vi "Big_LED_control.vi"() -> ()   [LabVIEW 2018]
uses:
  <instrlib>/niDCPower/nidcpower.llb/niDCPower Source Mode.ctl
  <instrlib>/niDCPower/nidcpower.llb/niDCPower Output Function.ctl
  AT lib/AmateurStepperMotor.dll
  <instrlib>/niDMM/nidmm.llb/niDMM Function.ctl
  <instrlib>/niDMM/nidmm.llb/niDMM Resolution in Digits.ctl
  <vilib>/Instr/_visa.llb/VISA Configure Serial Port (Instr).vi
  <instrlib>/niDMM/nidmm.llb/niDMM Configure Measurement Digits.vi
panel:
  in  "Tab Control 2":enum32{"Шаговик и офир", "Служебная область"}(tab)
  in  "milliseconds to wait":u32=1000
  in  "Go To":dbl
  out "Ophir 1 Char":dbl(graph)=0.02
  in  "DecelerationTime, s":dbl=0.3
  in  "AccelerationTime, s":dbl=0.3
  in  "HoldOn":bool
  in  "Ophir 1 units":string(combo)="1000" caption="Units"
  out "Ophir 1 Over Range":bool caption="Over Range"
  out "Ophir 1 Optical Power":dbl=0.02 caption="Power" format="%#_4g"
  out "Ophir 1 MAX":dbl=0.030000000000000002 caption="MAX" format="%#_5g"
  in  "Ophir 1 Clear":bool caption="Clear"
  in  "StepMultiplicationFactor":dbl=50.0
  in  "StepDivisor":i32(ring)=8 items=["D1"=1, "D2"=2, "D4"=4, "D8"=8, "D16"=16, "D32"=32]
  in  "Speed":dbl=250.0
  in  "Погнали!":bool
  in  "Стоп GoTo":bool
  out "Готово":bool
  out "Position":dbl
  in  "Ophir 1 Info":u16(ring)=1 caption="Info" items=["Device : JUNO; s/n:903793", "Head : PD300R-3W   ; s/n:779628"]
  in  "new pos":dbl
  in  "set pos":bool
  out "Device Response":string="*\n"
  in  "Ophir 1 usb channel":i16 caption="usb channel"
  out "Ophir 1 dup Visa Session":refnum<visa-resource-name>="USB0::0x0BD3::0x0777::NI-VISA-60004::RAW" caption="dup Visa Session"
  in  "Ophir 1 Baud Rate (3:9600)":i16(ring)=3 caption="Baud Rate (3:9600)" items=["300", "1200", "4800", "9600", "19200", "38400"]
  out "Ophir 1 Real Optical Power":dbl=2e-05 format="%.6e"
  in  "Ophir 1 GPIB Address (10)":string="10" caption="GPIB Address (10)"
  in  "Ophir 1 Port Number (default 2)":i16=1 caption="Port Number (default 2)" min=0 max=20
  in  "Ophir 1 Select Communication Protocol":u16(ring) caption="Select Communication Protocol" items=["USB", "RS232", "GPIB"]
  out "Ophir 1 error out":errorcluster caption="error out"
  in  "Ophir 1 error in (no error)":errorcluster caption="error in (no error)"
  in  "Ophir 1 Wait":u32=100 caption="Wait"
  out "IsOpen":bool=TRUE
  out "Ophir 1 Initialization":bool=TRUE caption="Initialization"
  in  "Tab Control":T1(tab)
  in  "POWER":bool
  in  "Стоп":bool=TRUE
  in  "Resource Name":refnum<k15>="PXI1Slot2" caption="Источник питания"
  in  "Амперметр":refnum<k15>="PXI1Slot4" caption="NI DMM 1"
  in  "V_MB, V":dbl=6.0 caption="voltage level" min=0.0 max=6.0 format="%_6p"
  in  "curlim_V_MB, A":dbl=0.3 caption="current limit" format="%_6p"
  out "chart_0":dbl(graph)=-0.00019003121552656476 caption="Waveform Chart 5"
  in  "voltlim_I_LED, V":dbl=2.1 caption="current limit" min=0.01 format="%_6p"
  in  "I_LED, A":dbl=0.010000000000000002 caption="voltage level" format="%_6p"
  out "chart_1":dbl(graph)=-0.00011794146773492402 caption="Waveform Chart 5"
  out "Current Char":dbl(graph)=0.004513189196586609
  in  "Arduino":refnum<visa-resource-name>="COM14"
  in  "Сегменты":bool[](array[boolean])=[FALSE, FALSE, FALSE, FALSE, FALSE, FALSE, FALSE, FALSE, FALSE, FALSE, FALSE, FALSE, FALSE, FALSE, FALSE, FALSE, FALSE, FALSE]
  in  "Вольтметр":refnum<k15>="PXI1Slot5" caption="NI DMM 1"
  out "Voltage Char":dbl(graph)=0.015767553821206093
  in  "Port Name":string="COM8" caption="Порт шаговика"
  in  "wave_lenght":string="600"
  in  "Промер":bool caption="Промер сегмента"
  in  "NI DMM 1 Voltage Range 4":string(combo)="-1" caption="Range"
  in  "NI DMM 1 units 4":string(combo)="1" caption="Units"
  out "Voltage":dbl=0.015767553821206093 format="%_6g"
  in  "NI DMM 1 Current Range 3":string(combo)="1" caption="Range"
  in  "NI DMM 1 units 3":string(combo)="1000" caption="Units"
  out "Current":dbl=0.004513189196586609 format="%_6g"
  out "voltmes_V_MB, V":dbl=-0.00019003121552656476 caption="measurement" format="%_6g"
  out "curmes_V_MB, A":dbl=4.978853713564661e-05 caption="measurement" format="%_6g"
  out "curmes_I_LED, A":dbl=4.978853713564661e-05 caption="measurement" format="%_6g"
  out "voltmes_I_LED, V":dbl=-0.00011794146773492402 caption="measurement" format="%_6g"
  out "Разряд":dbl
  out "+/-":bool
  out "Power off":bool=TRUE
  in  "Command":string="Cathode"
  in  "Записать":bool
  out "measure output \nfile refnum":refnum<file>
  out "Voltage, V":dbl=0.015767553821206093 caption="Measurement" format="%.5f"
  out "Current, A":dbl=4.513189196586609e-06 caption="Measurement" format="%.5f"
  out "Тип индикатора":string="Cathode"
  out "chart_2":dbl(graph)=-0.000179732680132088
  in  "V_RES, V":dbl caption="voltage level" format="%_6p"
  out "curmes_V_RES, A":dbl=5.996099535583298e-05 caption="measurement" format="%_6g"
  in  "curlim_V_RES, A":dbl=0.1 caption="current limit" min=0.01 format="%_6p"
  in  "measure path":path=path "C:/Users/user/Desktop/МСП/LabVIEW/LED_CONTROL_big_LED_ophir_24.12.24_1/Logs"
  out "Enum":enum16{"Exit", "4", "Промер", "2", "1"}(ring)
  out "№ об-ца":dbl=1.0
  out "Темп-ра":dbl=1.0
  out "Сегмент":string
  out "voltmes_V_RES, V":dbl=-0.000179732680132088 caption="measurement" format="%_6g"
  in  "current level range":dbl=0.001 format="%#.6p"
  # "При первом запуске  есть ошика при инициализации шаговика.\nПри втором запуске обишки нет, делать ничего не нужно.\n\nПоговорить с Артемом"
  # "Шаговик"
  # "Офир"
  # "Шаговик"
  # "Офир"
  # "position - это значение абсолютное"
  # "j"
  # "c"
  # "d"
  # "e"
  # "g"
  # "h"
  # "a"
  # "b"
  # "f"
  # "k"
  # "L"
  # "m"
  # "n"
  # "p"
  # "dp"
  # "all"
  # "V_MB 5 В\nогрничение 300 м\n\nV_LED 2,1 В\nограничение 200 м"
  # "единицы мА\nrange 1 А"
  # "1. каждый сегмент включаем по отдельности, резистором постраиваем ток до 10 мА\n2. напряжение V_LED при этом не меняется\n3. в такоом положении промеряем сегменты по отдельности\n4. для промера всего индикатора сразу подстраиваем напряжение при неизменном положении резисторов\n5. ток всех индикаторов = ток одного сегмента (10 мА) * число сегментов (15)\n6. добиваемся этого увеличением V_LED"
  # "единицы В\nrange AUTO"
  # "регклировка суммарного тока через индикатор"
  # "24.063\n\n     I          U\n20 мА  1.3 В\n20 мА  1.4 В\n 7 мА   1.15 В"
  # "24.064\n\n     I          U\n10 мА  2 В\n10 мА  2.15 В\n 7 мА   1.9 В"
  # "автоматизировать подбор напряжения по известному максимальному напряжению и току. ОС по току сегмента"
  # "Р1:  +25°C\nР2:  - 60°C\nР3:  +85°C"
  # "регулировать ток в зависимости от температуры.\nс ростом температуры растет ток.\nпид-регулятор??"
  # "0. ввести номер образца\n1. включить нужный сегмент\n2. ввести его в поле справа\n3. вести температуру в поле слева\n4. нажать кнопку \"промер сегмента\""
  # "\"опрашивать кнопки не чаще, чем раз в секунду. сейчас кликать можно чаще, они загорятся, но ничего не произойдет\""
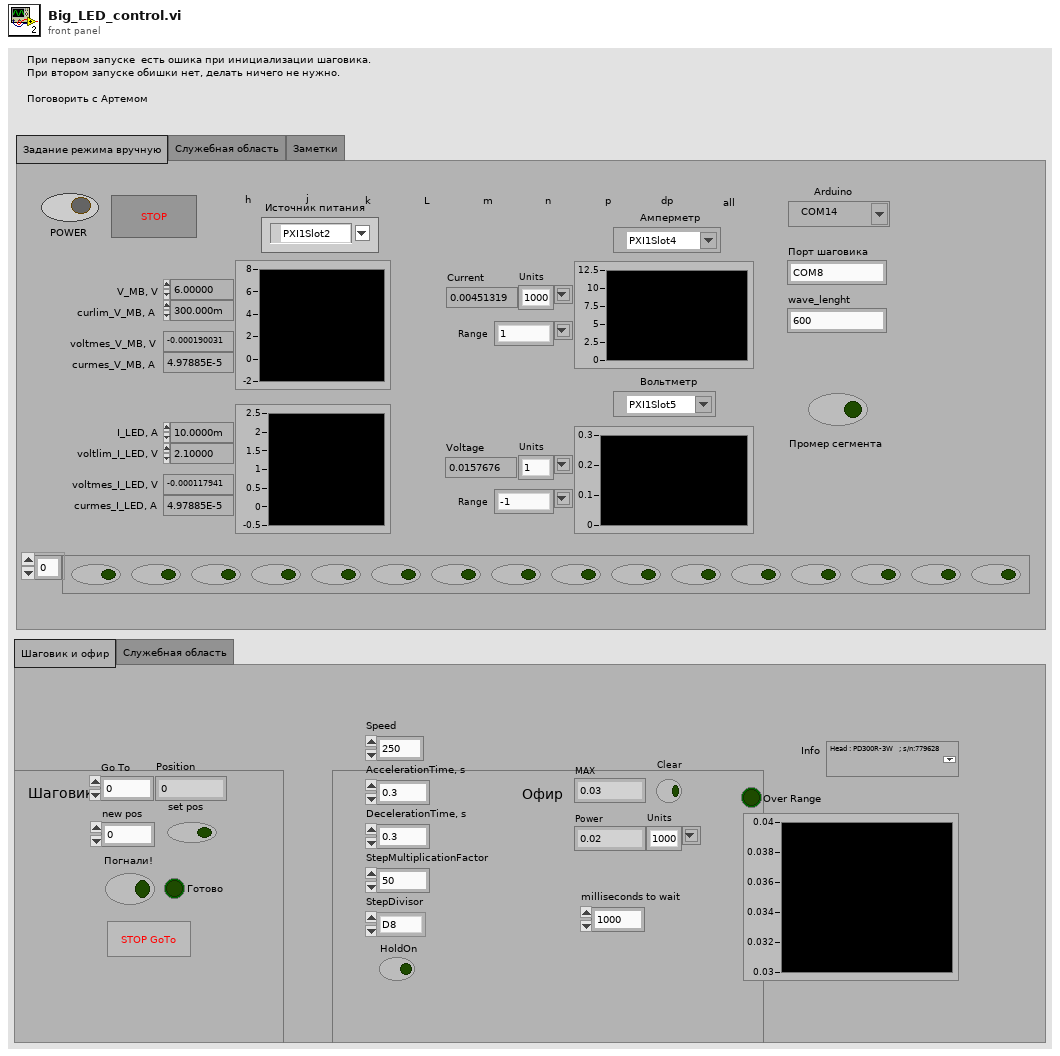
[diagram p1: front panel]
types:
  T1 = enum32{"Задание режима вручную", "Служебная область", "Заметки"}
  T2 = enum16{"open", "replace", "create", "open or create", "replace or create", "replace or create with confirmation"}
  T3 = typedef "niDCPower Output Function.ctl" = i32
  T4 = typedef "niDCPower Source Mode.ctl" = i32
  T5 = typedef "niDMM Function.ctl" = enum16{"DC Volts", "AC Volts", "DC Current", "AC Current", "2-wire Resistance", "4-wire Resistance", "Diode", "Frequency", "Period", "AC Volts DC Coupled", "Capacitance", "Inductance", "Temperature"}
  T6 = typedef "niDMM Resolution in Digits.ctl" = dbl
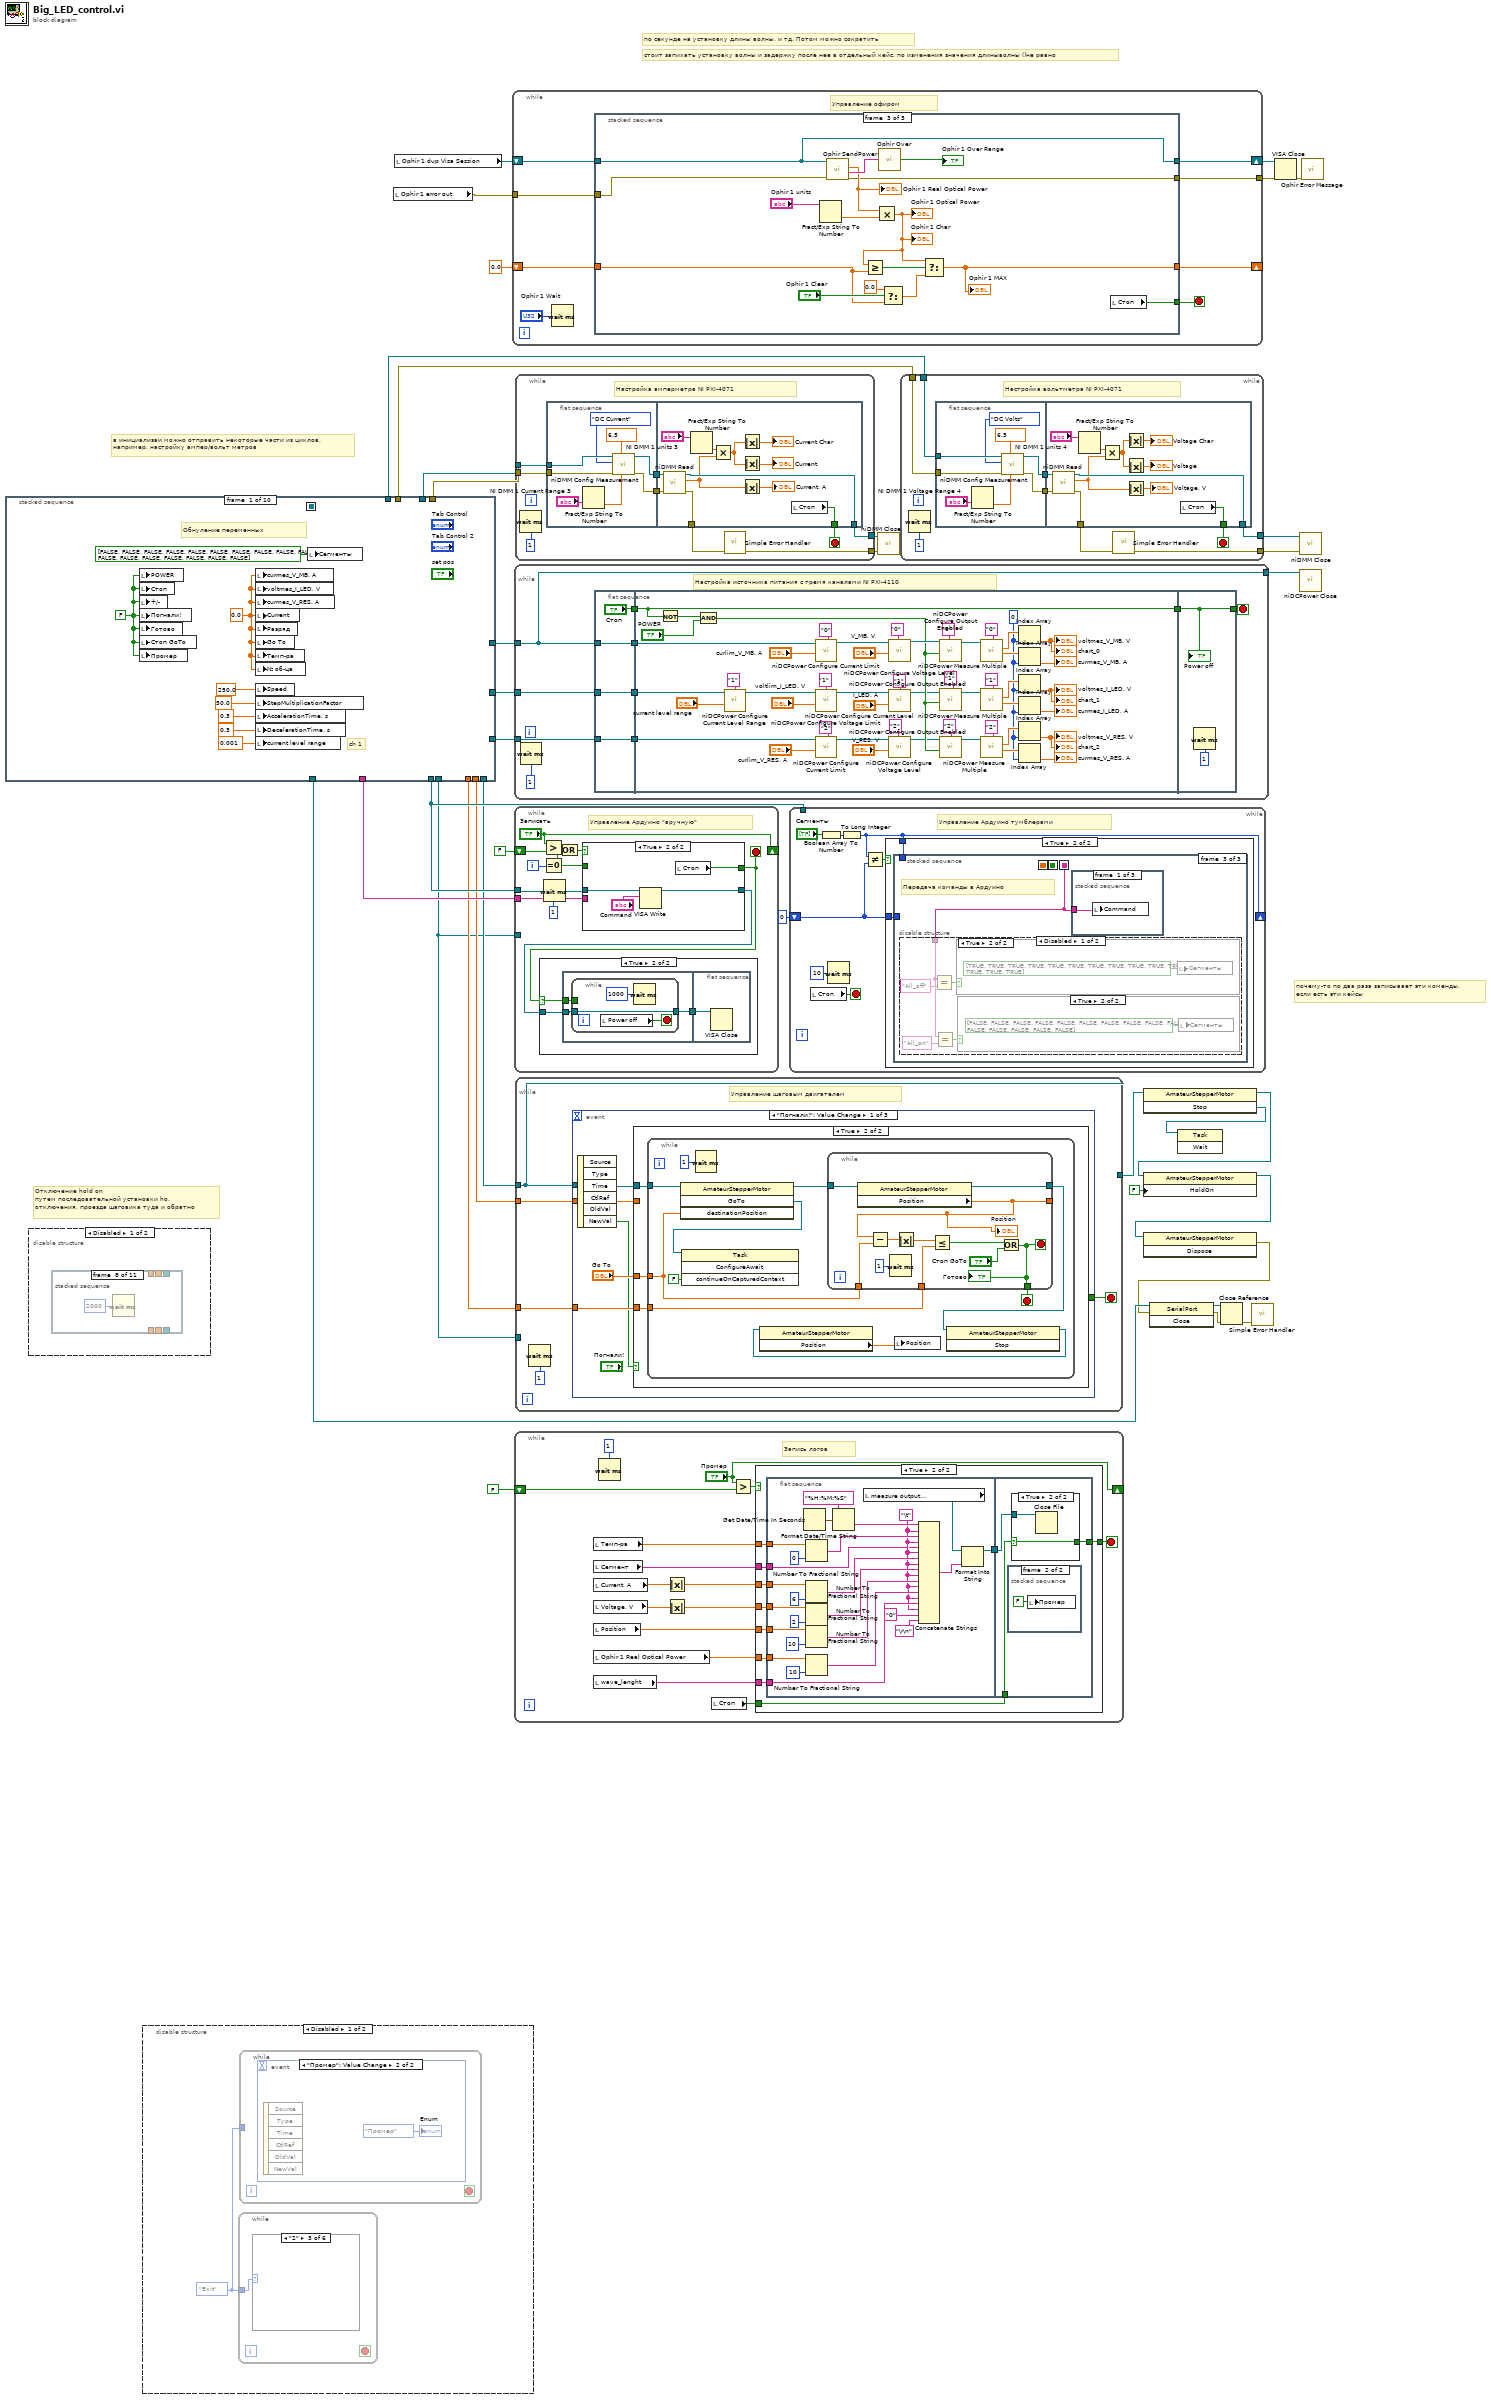
[diagram p0: block diagram]
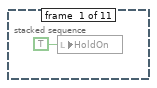
[diagram p2: hidden frame]
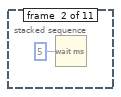
[diagram p3: hidden frame]
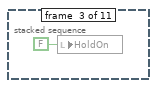
[diagram p4: hidden frame]
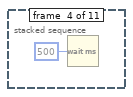
[diagram p5: hidden frame]
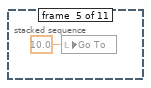
[diagram p6: hidden frame]
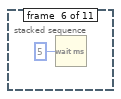
[diagram p7: hidden frame]
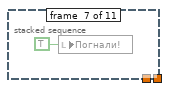
[diagram p8: hidden frame]
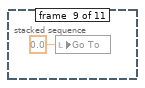
[diagram p9: hidden frame]
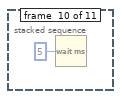
[diagram p10: hidden frame]
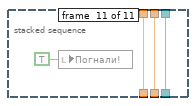
[diagram p11: hidden frame]
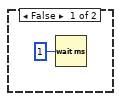
[diagram p13: hidden frame]
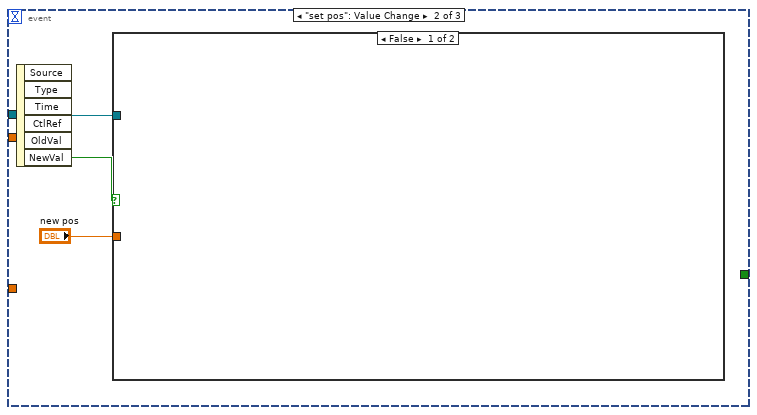
[diagram p14: hidden frame]
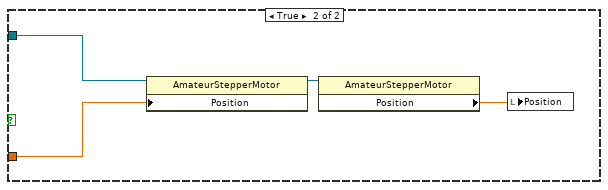
[diagram p15: hidden frame]
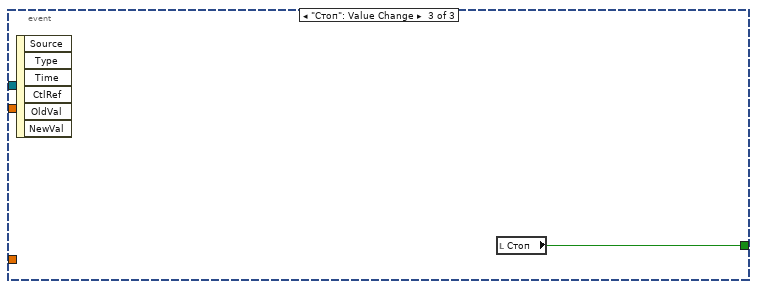
[diagram p16: hidden frame]
diagram:
  # "почему-то по два раза записывает эти коменды,\nесли есть эти кейсы"
  # "Отключение hold on\nпутем последовательной установки ho, \nотключения, проезда шаговика туда и обратно"
  # "в инициализаи можно отправить некоторые части из циклов.\nнапример, настройку ампер/вольт метров"
  # "стоит запихать установку волны и задержку после нее в отдельный кейс, по изменения значения длиныволны ()не равно"
  # "по секунде на установку длины волны, и тд. Потом можно сократить"
  n1 = stacked-sequence {
    seq-local: [_ _ _ _ _ _ w107 _ _ _] -> [_ _ _ _ _ _ _ w116 _ _]
    tunnel: [_ _ _ w54 _ _ _ _ _ _] -> w25
    tunnel: [_ w48 _ _ _ _ _ _ _ _] -> w37
    tunnel: [_ w47 _ _ _ _ _ _ _ _] -> w36
    tunnel: [_ _ _ _ w74 _ _ _ _ _] -> w33
    tunnel: [_ _ _ _ _ _ _ _ w122 _] -> w32
    tunnel: [_ _ w51 _ _ _ _ _ _ _] -> w31
    tunnel: [_ _ w50 _ _ _ _ _ _ _] -> w30
    tunnel: [_ _ _ _ _ _ _ w119 _ _] -> w2
    tunnel: [_ _ _ _ _ _ _ w117 _ _] -> w3
    tunnel: [_ _ _ _ _ _ _ w118 _ _] -> w4
    tunnel: [_ _ _ _ _ _ w97 _ _ _] -> w19
    tunnel: [_ _ _ w53 _ _ _ _ _ _] -> w7
    tunnel: [_ _ _ w52 _ _ _ _ _ _] -> w5
    tunnel: [_ _ _ _ _ _ _ _ _ w123] -> w1
    frame #0 {
      w38 = 0.0 ("currentmes_2")
      w39 = FALSE ("Стоп")
      # "ch 1"
      # "Обнуление переменных"
      n2 = local write "POWER"(w39) -> ()
      n3 = local write "Стоп"(w39) -> ()
      n4 = local write "+/-"(w39) -> ()
      n5 = local write "Погнали!"(w39) -> ()
      n6 = local write "Готово"(w39) -> ()
      n7 = local write "Стоп GoTo"(w39) -> ()
      n8 = local write "Промер"(w39) -> ()
      n9 = local write "curmes_V_MB, A"(w38) -> ()
      n10 = local write "voltmes_I_LED, V"(w38) -> ()
      n11 = local write "curmes_V_RES, A"(w38) -> ()
      n12 = local write "Current"(w38) -> ()
      n13 = local write "Разряд"(w38) -> ()
      n14 = local write "Go To"(w38) -> ()
      n15 = local write "Темп-ра"(w38) -> ()
      n16 = local write "№ об-ца"(w38) -> ()
      n17 = local write "Speed"(250.0 ("Speed")) -> ()
      n18 = local write "StepMultiplicationFactor"(50.0 ("StepMultiplicationFactor")) -> ()
      n19 = local write "AccelerationTime, s"(0.3 ("AccelerationTime, s")) -> ()
      n20 = local write "DecelerationTime, s"(0.3 ("DecelerationTime, s")) -> ()
      n21 = local write "current level range"(0.001 ("current level range")) -> ()
      n22 = local write "Сегменты"(bool[] [FALSE, FALSE, FALSE, FALSE, FALSE, FALSE, FALSE, FALSE, FALSE, FALSE, FALSE, FALSE, FALSE, FALSE, FALSE, FALSE, FALSE, FALSE] ("Сегменты")) -> ()
    }
    frame #1 {
      # "Инициализация амперметра"
      n23 = call <instrlib>:"niDMM Initialize.vi"("Instrument Descriptor"="Амперметр") -> ("error out"=w48:errorcluster, "instrument handle out"=w47:refnum<k15>)  [unwired: 9 in]
    }
    frame #2 {
      # "Инициализация вольтметра"
      n24 = call <instrlib>:"niDMM Initialize.vi"("Instrument Descriptor"="Вольтметр") -> ("error out"=w50:errorcluster, "instrument handle out"=w51:refnum<k15>)  [unwired: 9 in]
    }
    frame #3 {
      w59 = T3 1006 items=["DC Voltage"=1006, "DC Current"=1007, "Pulse Voltage"=1049, "Pulse Current"=1050] ("output function")
      w63 = T3 1007 items=["DC Voltage"=1006, "DC Current"=1007, "Pulse Voltage"=1049, "Pulse Current"=1050] ("output function")
      w64 = T3 1006 items=["DC Voltage"=1006, "DC Current"=1007, "Pulse Voltage"=1049, "Pulse Current"=1050] ("output function")
      w67 = T4 1020 items=["Single Point"=1020, "Sequence"=1021] ("source mode")
      # "Инициализация источника питания"
      n25 = call <instrlib>:"niDCPower Initialize.vi"("resource name"="Resource Name") -> ("instrument handle out"=w68:refnum<k15>)  [unwired: 3 in, 7 out]
      n26 = call <instrlib>:"niDCPower Configure Source Mode.vi"("source mode"=w67, "instrument handle"=w68) -> ("instrument handle out"=w58:refnum<k15>)  [unwired: 1 in, 8 out]
      n27 = call <instrlib>:"niDCPower Configure Output Function.vi"("output function"=w63, "channel name"="1", "instrument handle"=w58) -> ("instrument handle out"=w65:refnum<k15>)  [unwired: 7 in, 1 out]
      n28 = call <instrlib>:"niDCPower Configure Output Function.vi"("output function"=w59, "channel name"="2", "instrument handle"=w58) -> ("instrument handle out"=w60:refnum<k15>)  [unwired: 7 in, 1 out]
      n29 = call <instrlib>:"niDCPower Configure Output Function.vi"("output function"=w64, "channel name"="0", "instrument handle"=w58) -> ("instrument handle out"=w66:refnum<k15>)  [unwired: 7 in, 1 out]
      n30 = call <instrlib>:"niDCPower Configure Voltage Level.vi"("voltage level"=0.0, "channel name"="2", "instrument handle"=w60) -> ("instrument handle out"=w52:refnum<k15>)  [unwired: 7 in, 1 out]
      n31 = call <instrlib>:"niDCPower Configure Voltage Level.vi"("voltage level"=0.0, "channel name"="0", "instrument handle"=w66) -> ("instrument handle out"=w54:refnum<k15>)  [unwired: 7 in, 1 out]
      n32 = call <instrlib>:"niDCPower Configure Current Level.vi"("current level"=0.01, "channel name"="1", "instrument handle"=w65) -> ("instrument handle out"=w53:refnum<k15>)  [unwired: 7 in, 1 out]
    }
    frame #4 {
      # "Инициализация Ардуино"
      n33 = call-poly "VISA Configure Serial Port"("VISA resource name"="Arduino", "baud rate (9600)"=u32 9600) -> ("VISA resource name out"=w74:refnum<visa-resource-name>)  [unwired: 12 in, 1 out]
    }
    frame #5 {
      # "Инициализация офира"
      n34 = call "Ophir InitCom.vi"("GPIB Address (default 10)"="Ophir 1 GPIB Address (10)", "Communication (default USB 0)"="Ophir 1 Select Communication Protocol", "USB Channel number (default 0)"="Ophir 1 usb channel", "Port Number (default 2)"="Ophir 1 Port Number (default 2)", "error in (no error)"="Ophir 1 error in (no error)", "Baud Rate (3:9600)"="Ophir 1 Baud Rate (3:9600)") -> ("dup Visa Session"=w83:refnum<visa-resource-name>, "error out"=w82:errorcluster)  [unwired: 1 out]
      n35 = call "Ophir InstrInfo.vi"("Visa Session"=w83, "error in (no error)"=w82) -> ("dup Visa Session"=w95:refnum<visa-resource-name>, "Instrument Info"=w77:string, "error out"=w93:errorcluster)
      n36 = call "Ophir HeadInfo.vi"("Visa Session"=w95, "error in (no error)"=w93) -> ("error out"=w92:errorcluster, "dup Visa Session"=w94:refnum<visa-resource-name>, "Head Info"=w91:string)  [unwired: 6 out]
      n37 = call "Ophir InfoStrings.vi"("error in (no error)"=w92, "Head Info"=w91, "Instrument Info"=w77) -> ("error out"=w90:errorcluster, "Strings Array"=w89:string[])
      n38 = property on="Ophir 1 Info" class="Ring (strict)"("Strings []"=w89) -> ()  [unwired: 2 in, 2 out]
      n39 = call "Ophir ConfigDevice.vi"("Visa Session"=w94, "Measure Choice (0:Power)"=u16 0, "error in (no error)"=w90) -> ("dup Visa Session"=→"Ophir 1 dup Visa Session":refnum<visa-resource-name>, "OK ?"=→"Ophir 1 Initialization":bool, "error out"=→"Ophir 1 error out":errorcluster)  [unwired: 1 out]
    }
    frame #6 {
      w101 = 100 ("WriteTimeout")
      w106 = 1 items=["None", "One", "Two", "OnePointFive"] ("stopBits")
      w103 = 0 items=["None", "Odd", "Even", "Mark", "Space"] ("parity")
      # "убрали открытие порта. шаговик его и так сам откроет"
      # "Инициализация шаговика ч.1"
      n40 = constructor class="SerialPort"("portName"="Port Name", "baudRate"=57600, "parity"=w103, "dataBits"=8, "stopBits"=w106) -> (reference out=w100:refnum<k24>, error out=w99:errorcluster)  [unwired: 3 in, 6 out]
      n41 = property class="SerialPort"(reference=w100, error in=w99, "WriteTimeout"=w101, "ReadTimeout"=w101) -> (reference out=w97:refnum<k24>)  [unwired: 1 out]
      n42 = constructor class="AmateurStepperMotor"("serialPort"=w97) -> (reference out=w107:refnum<k24>, error out=w98:errorcluster)  [unwired: 3 in, 2 out]
      n43 = flat-sequence {
        tunnel: w98 -> [_]
        tunnel: w97 -> [w109]
        frame #0 {
          n44 = property class="SerialPort"(reference=w109) -> ("IsOpen"=→"IsOpen":bool)  [unwired: 1 in, 2 out]
        }
      }
    }
    frame #7 {
      # "стоит допустить изменение\nтих параметров в цикле, а не только \nпри инициализации"
      # "это те самые 50 шагов за мм"
      # "Инициализация шаговика ч.2"
      n45 = property class="AmateurStepperMotor"(reference=w116, "Speed"="Speed", "StepDivisor"="StepDivisor", "StepMultiplicationFactor"="StepMultiplicationFactor", "AccelerationTime"="AccelerationTime, s", "DecelerationTime"="DecelerationTime, s", "HoldOn"="HoldOn") -> (reference out=w119:refnum<k24>, "Position"=w117:dbl, "PositioningPrecision"=w118:dbl)  [unwired: 1 in, 1 out]
    }
    frame #8 {
      # "Begin VI: ОК или ОА?"
      n46 = call "Begin.vi"() -> ("Темп-ра"=→"Темп-ра":dbl, "№ об-ца"=→"№ об-ца":dbl, "String"=w122:string)  [unwired: 6 in]
      "Тип индикатора" <- w122
      n47 = local write "Command"(w122) -> ()
    }
    frame #9 {
      w133 = "\t"
      # "Инициализация логов"
      n48 = local read "№ об-ца"() -> (w137:dbl)
      n49 = Number To Fractional String(number=w137, precision (6)=i16 0) -> (F-format string=w138:string)  [unwired: 2 in]
      n50 = Get Date/Time In Seconds() -> (seconds since 1Jan1904=w148:timestamp)
      n51 = Build Path(base path="measure path", name or relative path=w138) -> (appended path=w144:path)
      n52 = call <vilib>:"Check if File or Folder Exists.vi"("path"=w144) -> ("file or folder exists?"=w145:bool, "dup path"=w146:path)  [unwired: 8 in, 1 out]
      n53 = Format Date/Time String(time format string (%c)="MES %d. %m. %y %H.%M.%S", seconds (now)=w148) -> (date/time string=w149:string)  [unwired: 1 in]
      n54 = case shown="True" w145 {
        tunnel: w146 -> [w155 w156]
        tunnel: [w154 w156] -> w147
        frame False {
          n55 = Create Folder(path (use dialog)=w155) -> (created path=w154:path)  [unwired: 2 in, 2 out]
        }
        frame True {
        }
      }
      n56 = Concatenate Strings(w149, ".xls" ("string")) -> (w150:string)
      n57 = Build Path(base path=w147, name or relative path=w150) -> (appended path=w151:path)
      n58 = Open/Create/Replace File(file path (use dialog)=w151, operation (0:open)=T2."open or create", access (0:read/write)=enum16{"read/write", "read-only", "write-only"}."read/write") -> (refnum out=w152:refnum<file>)  [unwired: 3 in, 2 out]
      n59 = Set File Position(refnum=w152, from (0:start)=enum16{"start", "end", "current"}."end") -> (refnum out=w135:refnum<file>)  [unwired: 2 in, 1 out]
      n60 = Format Into String(initial string=w135, "Time" ("string"), w133, "Temperature, C" ("string"), w133, "Segment" ("string"), w133, "Current, mA" ("string"), w133, "Voltage, V" ("input 7"), w133, "Distance, m" ("string"), w133, "Power, W " ("string"), w133, "Wavelenght, nm" ("input 17"), w133, "Candlepower, kd" ("string"), "\r\n") -> (resulting string=w123:refnum<file>)  [unwired: 2 in, 1 out]
      "measure output \nfile refnum" <- w123
    }
  }
  n61 = disable-structure shown="Disabled" {
    frame Disabled {
      n62 = stacked-sequence {
        tunnel: _ -> [_ _ _ _ _ _ _ _ _ _ w169]
        tunnel: [_ _ _ _ _ _ _ _ _ _ w169] -> _
        tunnel: _ -> [_ _ _ _ _ _ _ _ _ _ w168]
        tunnel: [_ _ _ _ _ _ _ _ _ _ w168] -> _
        tunnel: [_ _ _ _ _ _ _ _ _ _ w167] -> _
        tunnel: _ -> [_ _ _ _ _ _ _ _ _ _ w167]
        frame #0 {
          n63 = local write "HoldOn"(TRUE ("HoldOn")) -> ()
        }
        frame #1 {
          n64 = Wait (ms)(milliseconds to wait=u32 5) -> ()  [unwired: 1 out]
        }
        frame #2 {
          n65 = local write "HoldOn"(FALSE ("HoldOn")) -> ()
        }
        frame #3 {
          n66 = Wait (ms)(milliseconds to wait=u32 500) -> ()  [unwired: 1 out]
        }
        frame #4 {
          n67 = local write "Go To"(10.0 ("Go To")) -> ()
        }
        frame #5 {
          n68 = Wait (ms)(milliseconds to wait=u32 5) -> ()  [unwired: 1 out]
        }
        frame #6 {
          n69 = local write "Погнали!"(TRUE ("Погнали!")) -> ()
        }
        frame #7 {
          n70 = Wait (ms)(milliseconds to wait=u32 2000) -> ()  [unwired: 1 out]
        }
        frame #8 {
          n71 = local write "Go To"(0.0 ("Go To")) -> ()
        }
        frame #9 {
          n72 = Wait (ms)(milliseconds to wait=u32 5) -> ()  [unwired: 1 out]
        }
        frame #10 {
          n73 = local write "Погнали!"(TRUE ("Погнали!")) -> ()
        }
      }
    }
    frame Enabled {
    }
  }
  n74 = disable-structure shown="Disabled" {
    frame Disabled {
      w171 = enum16{"Exit", "4", "Промер", "2", "1"}."Exit"
      n75 = while {
        tunnel: w171 -> [w172]
        stop <- _ stop-if-true
        n76 = case shown="\"2\"" w172 {
          frame "Exit", Default {
          }
          frame "4" {
          }
          frame "2" {
          }
          frame "2" {
          }
          frame "1" {
          }
          frame "Промер" {
          }
        }
      }
      n77 = while {
        tunnel: w171 -> [_]
        stop <- _ stop-if-true
        n78 = event shown="[1] \"Промер\": Value Change" {
          selector: _ -> [_ _]
          dyn-events: _ -> [_ _]
          timeout: _ -> [_ _]
          event Timeout {
            n79 = event-data() -> ()  [unwired: 1 in, 3 out]
          }
          event "Промер": Value Change {
            n80 = event-data() -> ()  [unwired: 1 in, 6 out]
            "Enum" <- enum16{"Exit", "4", "Промер", "2", "1"}."Промер" ("Enum")
          }
        }
      }
    }
    frame Enabled {
    }
  }
  n81 = local read "Ophir 1 error out"() -> (w23:errorcluster)
  n82 = local read "Ophir 1 dup Visa Session"() -> (w24:refnum<visa-resource-name>)
  n83 = while {
    tunnel: w23 -> [w180]
    shift-right: [w176] -> _
    shift-left: 0.0 ("t") -> [w179]
    shift-right: [w177] -> w17
    shift-left: w24 -> [w181]
    tunnel: [w175] -> w16
    stop <- w174 stop-if-true
    # "Управление офиром"
    n84 = Wait (ms)(milliseconds to wait="Ophir 1 Wait") -> ()  [unwired: 1 out]
    n85 = stacked-sequence {
      tunnel: w181 -> [w185 _ w188]
      tunnel: w180 -> [w184 _ w190]
      tunnel: w179 -> [_ _ w191]
      tunnel: [_ _ w188] -> w177
      tunnel: [_ _ w192] -> w176
      tunnel: [_ _ w189] -> w175
      tunnel: [_ _ w187] -> w174
      frame #0 {
        n86 = call "light_setWaveLenght.vi"("error in (no error)"=w184, "Visa Session"=w185, "wave_lenght"="wave_lenght") -> ("Device Response"=→"Device Response":string)  [unwired: 6 in, 2 out]
      }
      frame #1 {
        n87 = Wait (ms)(milliseconds to wait="milliseconds to wait") -> ()  [unwired: 1 out]
      }
      frame #2 {
        n88 = Fract/Exp String To Number(string="Ophir 1 units") -> (number=w195:dbl)  [unwired: 3 in, 1 out]
        n89 = call "Ophir SendPower.vi"("Visa Session"=w188, "error in (no error)"=w190) -> ("Value Number"=w194:dbl, "Value String"=w201:string, "error out"=w189:errorcluster)  [unwired: 1 out]
        "Ophir 1 Real Optical Power" <- w194
        n90 = Multiply(x=w194, y=w195) -> (x*y=w198:dbl)
        "Ophir 1 Char" <- w198
        "Ophir 1 Optical Power" <- w198
        n91 = Greater Or Equal?(x=w198, y=w191) -> (x >= y?=w199:bool)
        n92 = call "Ophir Over.vi"("Value String"=w201) -> ("Overrange"=→"Ophir 1 Over Range":bool)
        n93 = Select(t=0.0, s="Ophir 1 Clear", f=w191) -> (s? t:f=w197:dbl)
        n94 = Select(t=w198, s=w199, f=w197) -> (s? t:f=w192:dbl)
        "Ophir 1 MAX" <- w192
        n95 = local read "Стоп"() -> (w187:bool)
      }
    }
  }
  n96 = while {
    tunnel: w25 -> [w209]
    tunnel: [w209] -> w34
    tunnel: w7 -> [w206]
    tunnel: w5 -> [w203]
    stop <- w205 stop-if-true
    # "Настройка источника питания с тремя каналами NI PXI-4110"
    n97 = Wait (ms)(milliseconds to wait=u32 1) -> ()  [unwired: 1 out]
    n98 = flat-sequence {
      tunnel: w209 -> [w216]
      tunnel: [w216] -> w211
      tunnel: ["Стоп"] -> w210
      tunnel: [w214] -> w207
      tunnel: w206 -> [w214]
      tunnel: [w213] -> w204
      tunnel: w203 -> [w213]
      tunnel: w211 -> [w262]
      tunnel: w210 -> [w266]
      tunnel: [w266] -> w208
      tunnel: w207 -> [w230]
      tunnel: w204 -> [w223]
      tunnel: [w268] -> w205
      tunnel: w208 -> [w268]
      frame #0 {
      }
      frame #1 {
        w231 = 0 ("index")
        n99 = Not(x=w266) -> (.not. x?=w265:bool)
        n100 = And(x=w265, y="POWER") -> (x .and. y?=w261:bool)
        n101 = call <instrlib>:"niDCPower Configure Current Level Range.vi"("current level range"="current level range", "channel name"="1", "instrument handle"=w230) -> ("instrument handle out"=w229:refnum<k15>)  [unwired: 7 in, 1 out]
        n102 = call <instrlib>:"niDCPower Configure Current Limit.vi"("current limit"="curlim_V_MB, A", "channel name"="0", "instrument handle"=w262) -> ("instrument handle out"=w252:refnum<k15>)  [unwired: 7 in, 1 out]
        n103 = call <instrlib>:"niDCPower Configure Voltage Limit.vi"("voltage limit"="voltlim_I_LED, V", "channel name"="1", "instrument handle"=w229) -> ("instrument handle out"=w256:refnum<k15>)  [unwired: 7 in, 1 out]
        n104 = call <instrlib>:"niDCPower Configure Current Limit.vi"("current limit"="curlim_V_RES, A", "channel name"="2", "instrument handle"=w223) -> ("instrument handle out"=w246:refnum<k15>)  [unwired: 7 in, 1 out]
        n105 = call <instrlib>:"niDCPower Configure Voltage Level.vi"("voltage level"="V_MB, V", "channel name"="0", "instrument handle"=w252) -> ("instrument handle out"=w263:refnum<k15>)  [unwired: 7 in, 1 out]
        n106 = call <instrlib>:"niDCPower Configure Current Level.vi"("current level"="I_LED, A", "channel name"="1", "instrument handle"=w256) -> ("instrument handle out"=w257:refnum<k15>)  [unwired: 7 in, 1 out]
        n107 = call <instrlib>:"niDCPower Configure Voltage Level.vi"("voltage level"="V_RES, V", "channel name"="2", "instrument handle"=w246) -> ("instrument handle out"=w247:refnum<k15>)  [unwired: 7 in, 1 out]
        n108 = call <instrlib>:"niDCPower Configure Output Enabled.vi"("output enabled"=w261, "channel name"="0", "instrument handle"=w263) -> ("instrument handle out"=w240:refnum<k15>)  [unwired: 7 in, 1 out]
        n109 = call <instrlib>:"niDCPower Configure Output Enabled.vi"("output enabled"=w261, "channel name"="1", "instrument handle"=w257) -> ("instrument handle out"=w233:refnum<k15>)  [unwired: 7 in, 1 out]
        n110 = call <instrlib>:"niDCPower Configure Output Enabled.vi"("output enabled"=w261, "channel name"="2", "instrument handle"=w247) -> ("instrument handle out"=w232:refnum<k15>)  [unwired: 7 in, 1 out]
        n111 = call <instrlib>:"niDCPower Measure Multiple.vi"("channel name"="0", "instrument handle"=w240) -> ("current measurements"=w238:dbl[], "voltage measurements"=w239:dbl[])  [unwired: 6 in, 2 out]
        n112 = call <instrlib>:"niDCPower Measure Multiple.vi"("channel name"="1", "instrument handle"=w233) -> ("current measurements"=w236:dbl[], "voltage measurements"=w237:dbl[])  [unwired: 6 in, 2 out]
        n113 = call <instrlib>:"niDCPower Measure Multiple.vi"("channel name"="2", "instrument handle"=w232) -> ("current measurements"=w234:dbl[], "voltage measurements"=w235:dbl[])  [unwired: 6 in, 2 out]
        n114 = Index Array(array=w239, index=w231) -> (element=→"chart_0" →"voltmes_V_MB, V":dbl)
        n115 = Index Array(array=w238, index=w231) -> (element=→"curmes_V_MB, A":dbl)
        n116 = Index Array(array=w237, index=w231) -> (element=→"chart_1" →"voltmes_I_LED, V":dbl)
        n117 = Index Array(array=w236, index=w231) -> (element=→"curmes_I_LED, A":dbl)
        n118 = Index Array(array=w235, index=w231) -> (element=→"chart_2" →"voltmes_V_RES, V":dbl)
        n119 = Index Array(array=w234, index=w231) -> (element=→"curmes_V_RES, A":dbl)
      }
      frame #2 {
        n120 = Wait (ms)(milliseconds to wait=u32 1) -> ()  [unwired: 1 out]
        "Power off" <- w268
      }
    }
  }
  n121 = while {
    tunnel: w33 -> [w276]
    shift-right: ["Записать"] -> _
    shift-left: FALSE ("Записать") -> [w278]
    tunnel: w32 -> [w274]
    tunnel: w1 -> [_]
    i -> [w275]
    stop <- w269 stop-if-true
    # "Управление Ардуино \"вручную\""
    n122 = Greater?(x="Записать", y=w278) -> (0:w272:bool)
    n123 = Equal To 0?(x=w275) -> (x = 0?=w271:bool)
    n124 = Wait (ms)(milliseconds to wait=u32 1) -> ()  [unwired: 1 out]
    n125 = Or(x=w272, y=w271) -> (x .or. y?=w273:bool)
    n126 = case shown="True" w273 {
      tunnel: w276 -> [w290 w295]
      tunnel: [w291 w294] -> w269
      tunnel: w274 -> [_ _]
      tunnel: w271 -> [_ _]
      tunnel: [w290 w292] -> w270
      frame False {
        n127 = local read "Стоп"() -> (w291:bool)
      }
      frame True {
        n128 = VISA Write(VISA resource name=w295, write buffer="Command") -> (VISA resource name out=w292:refnum<visa-resource-name>)  [unwired: 1 in, 2 out]
        n129 = local read "Стоп"() -> (w294:bool)
      }
    }
    n130 = case shown="True" w269 {
      selector: w269 -> [_ w280]
      tunnel: w270 -> [_ w282]
      frame False {
      }
      frame True {
        n131 = flat-sequence {
          tunnel: w282 -> [w285]
          tunnel: [w284] -> w281
          tunnel: w280 -> [w283]
          tunnel: w281 -> [w289]
          frame #0 {
            n132 = while {
              tunnel: w285 -> [w288]
              tunnel: [w288] -> w284
              tunnel: w283 -> [_]
              stop <- w286 stop-if-true
              n133 = local read "Power off"() -> (w286:bool)
              n134 = Wait (ms)(milliseconds to wait=u32 1000) -> ()  [unwired: 1 out]
            }
          }
          frame #1 {
            n135 = VISA Close(VISA resource name=w289) -> ()  [unwired: 1 in, 1 out]
          }
        }
      }
    }
  }
  n136 = while {
    shift-right: ["Промер"] -> _
    shift-left: FALSE ("Промер сегмента") -> [w308]
    stop <- w305 stop-if-true
    # "Запиcь логов"
    n137 = local read "Темп-ра"() -> (w301:dbl)
    n138 = local read "Сегмент"() -> (w302:string)
    n139 = local read "Current, A"() -> (w304:dbl)
    n140 = local read "Voltage, V"() -> (w303:dbl)
    n141 = local read "Position"() -> (w300:dbl)
    n142 = local read "Ophir 1 Real Optical Power"() -> (w298:dbl)
    n143 = local read "wave_lenght"() -> (w299:string)
    n144 = Wait (ms)(milliseconds to wait=u32 1) -> ()  [unwired: 1 out]
    n145 = Absolute Value(x=w304) -> (abs(x)=w296:dbl)
    n146 = Absolute Value(x=w303) -> (abs(x)=w297:dbl)
    n147 = local read "Стоп"() -> (w306:bool)
    n148 = Greater?(x="Промер", y=w308) -> (0:w309:bool)
    n149 = case shown="True" w309 {
      tunnel: w296 -> [_ w321]
      tunnel: w297 -> [_ w320]
      tunnel: w300 -> [_ w317]
      tunnel: w298 -> [_ w318]
      tunnel: w299 -> [_ w319]
      tunnel: w306 -> [w311 w315]
      tunnel: w301 -> [_ w314]
      tunnel: w302 -> [_ w313]
      tunnel: [w311 w312] -> w305
      frame False {
      }
      frame True {
        n150 = flat-sequence {
          tunnel: w321 -> [w339]
          tunnel: w320 -> [w338]
          tunnel: w319 -> [w336]
          tunnel: w318 -> [w335]
          tunnel: w317 -> [w334]
          tunnel: [w329] -> w316
          tunnel: w314 -> [w328]
          tunnel: w313 -> [w322]
          tunnel: w316 -> [w350]
          tunnel: w315 -> [w349]
          tunnel: [w348] -> w312
          frame #0 {
            w324 = "\t"
            n151 = Get Date/Time In Seconds() -> (seconds since 1Jan1904=w347:timestamp)
            n152 = Number To Fractional String(number=w328, precision (6)=i16 0) -> (F-format string=w326:string)  [unwired: 2 in]
            n153 = Number To Fractional String(number=w339, precision (6)=i16 6) -> (F-format string=w342:string)  [unwired: 2 in]
            n154 = Number To Fractional String(number=w338, precision (6)=i16 2) -> (F-format string=w341:string)  [unwired: 2 in]
            n155 = Number To Fractional String(number=w334, precision (6)=i16 10) -> (F-format string=w340:string)  [unwired: 2 in]
            n156 = Number To Fractional String(number=w335, precision (6)=i16 10) -> (F-format string=w337:string)  [unwired: 2 in]
            n157 = Format Date/Time String(time format string (%c)="%H:%M:%S", seconds (now)=w347) -> (date/time string=w345:string)  [unwired: 1 in]
            n158 = local read "measure output \nfile refnum"() -> (w343:refnum<file>)
            n159 = Concatenate Strings(w345, w324, w326, w324, w322, w324, w342, w324, w341, w324, w340, w324, w337, w324, w336, w324, "0" ("string"), "\r\n") -> (w344:string)
            n160 = Format Into String(initial string=w343, w344) -> (resulting string=w329:refnum<file>)  [unwired: 2 in, 1 out]
          }
          frame #1 {
            n161 = stacked-sequence {
              frame #0 {
                n162 = Wait (ms)(milliseconds to wait=u32 250) -> ()  [unwired: 1 out]
              }
              frame #1 {
                n163 = local write "Промер"(FALSE ("Промер")) -> ()
              }
            }
            n164 = case shown="True" w349 {
              selector: w349 -> [_ w354]
              tunnel: w350 -> [_ w355]
              tunnel: [FALSE w354] -> w348
              frame False {
              }
              frame True {
                n165 = Close File(refnum=w355) -> ()  [unwired: 1 in, 2 out]
              }
            }
          }
        }
      }
    }
  }
  n166 = while {
    tunnel: [w362] -> w26
    tunnel: w36 -> [w360]
    tunnel: w37 -> [w359]
    tunnel: [w356] -> w27
    stop <- w358 stop-if-true
    # "Настройка амперметра NI PXI-4071"
    n167 = Wait (ms)(milliseconds to wait=u32 1) -> ()  [unwired: 1 out]
    n168 = flat-sequence {
      tunnel: [w369] -> w364
      tunnel: w360 -> [w367]
      tunnel: w359 -> [w371]
      tunnel: [w368] -> w363
      tunnel: w364 -> [w381]
      tunnel: w363 -> [w384]
      tunnel: [w380] -> w358
      tunnel: [w379] -> w356
      tunnel: [w378] -> w357
      frame #0 {
        w365 = T6 6.5 items=["3 1/2"=3.5, "4 1/2"=4.5, "5 1/2"=5.5, "6 1/2"=6.5, "7 1/2"=7.5] ("Resolution in Digits")
        n169 = Fract/Exp String To Number(string="NI DMM 1 Current Range 3") -> (number=w370:dbl)  [unwired: 3 in, 1 out]
        n170 = call-poly <instrlib>:"niDMM Config Measurement.vi"("Range"=w370, "Resolution in Digits"=w365, "error in (no error)"=w371, "Function"=niDMM_Function."DC Current" ("Measurement Type"), "instrument handle"=w367) -> ("error out"=w368:errorcluster, "instrument handle out"=w369:refnum<k15>)  [unwired: 5 in]
      }
      frame #1 {
        n171 = call <instrlib>:"niDMM Read.vi"("error in (no error)"=w384, "instrument handle"=w381) -> ("error out"=w378:errorcluster, "Measurement"=w373:dbl, "instrument handle out"=w379:refnum<k15>)  [unwired: 7 in]
        n172 = Fract/Exp String To Number(string="NI DMM 1 units 3") -> (number=w382:dbl)  [unwired: 3 in, 1 out]
        n173 = Multiply(x=w382, y=w373) -> (x*y=w375:dbl)
        n174 = Absolute Value(x=w375) -> (abs(x)=→"Current Char":dbl)
        n175 = Absolute Value(x=w375) -> (abs(x)=→"Current":dbl)
        n176 = Absolute Value(x=w373) -> (abs(x)=→"Current, A":dbl)
        n177 = local read "Стоп"() -> (w380:bool)
      }
    }
    n178 = call <vilib>:"Simple Error Handler.vi"("error in (no error)"=w357) -> ("error out"=w362:errorcluster)  [unwired: 1 in, 7 out]
  }
  n179 = while {
    tunnel: w2 -> [w386]
    tunnel: w4 -> [w388]
    tunnel: [w386] -> w6
    tunnel: w3 -> [w389]
    tunnel: w1 -> [_]
    stop <- w385 stop-if-true
    # "Управление шаговым двигателем"
    n180 = Wait (ms)(milliseconds to wait=u32 1) -> ()  [unwired: 1 out]
    n181 = event shown="[0] \"Погнали!\": Value Change" {
      selector: _ -> [_ _ _]
      dyn-events: _ -> [_ _ _]
      timeout: _ -> [_ _ _]
      tunnel: w386 -> [w394 w422 _]
      tunnel: w389 -> [w393 _ _]
      tunnel: w388 -> [w392 _ _]
      tunnel: [_ _ w428] -> w385
      event "Погнали!": Value Change {
        n182 = event-data() -> ("NewVal"=w390:bool)  [unwired: 1 in, 5 out]
        n183 = case shown="True" w390 {
          tunnel: "Go To" -> [_ w398]
          tunnel: w394 -> [_ w397]
          tunnel: w393 -> [_ _]
          tunnel: w392 -> [_ w396]
          frame False {
            n184 = Wait (ms)(milliseconds to wait=u32 1) -> ()  [unwired: 1 out]
          }
          frame True {
            n185 = while {
              tunnel: w398 -> [w405]
              tunnel: w397 -> [w406]
              tunnel: w396 -> [w408]
              stop <- w409 stop-if-true
              n186 = invoke class="AmateurStepperMotor" method="GoTo"(reference=w406, "destinationPosition"=w405) -> (reference out=w401:refnum<k24>, "GoTo"=w404:refnum<k24>)  [unwired: 2 in, 2 out]
              n187 = invoke class="Task" method="ConfigureAwait"(reference=w404, "continueOnCapturedContext"=FALSE) -> ()  [unwired: 2 in, 4 out]
              n188 = Wait (ms)(milliseconds to wait=u32 1) -> ()  [unwired: 1 out]
              n189 = while {
                tunnel: [w410] -> _
                tunnel: [w412] -> w402
                tunnel: [w414] -> w409
                tunnel: w405 -> [w419]
                tunnel: w408 -> [w417]
                tunnel: w401 -> [w411]
                stop <- w414 stop-if-true
                n190 = property class="AmateurStepperMotor"(reference=w411) -> (reference out=w412:refnum<k24>, "Position"=w410:dbl)  [unwired: 1 in, 1 out]
                "Position" <- w410
                n191 = Subtract(x=w410, y=w419) -> (x-y=w420:dbl)
                n192 = Wait (ms)(milliseconds to wait=u32 1) -> ()  [unwired: 1 out]
                n193 = Absolute Value(x=w420) -> (abs(x)=w418:dbl)
                n194 = Less Or Equal?(x=w418, y=w417) -> (x <= y?=w416:bool)
                n195 = Or(x=w416, y="Стоп GoTo") -> (x .or. y?=w414:bool)
                "Готово" <- w414
              }
              n196 = invoke class="AmateurStepperMotor" method="Stop"(reference=w402) -> (reference out=w400:refnum<k24>)  [unwired: 2 in, 2 out]
              n197 = property class="AmateurStepperMotor"(reference=w400) -> ("Position"=w399:dbl)  [unwired: 1 in, 2 out]
              n198 = local write "Position"(w399) -> ()
            }
          }
        }
      }
      event "set pos": Value Change {
        n199 = event-data() -> ("NewVal"=w423:bool)  [unwired: 1 in, 5 out]
        n200 = case shown="False" w423 {
          tunnel: w422 -> [_ w427]
          tunnel: "new pos" -> [_ w426]
          frame False {
          }
          frame True {
            n201 = property class="AmateurStepperMotor"(reference=w427, "Position"=w426) -> (reference out=w425:refnum<k24>)  [unwired: 1 in, 1 out]
            n202 = property class="AmateurStepperMotor"(reference=w425) -> ("Position"=w424:dbl)  [unwired: 1 in, 2 out]
            n203 = local write "Position"(w424) -> ()
          }
        }
      }
      event "Стоп": Value Change {
        n204 = event-data() -> ()  [unwired: 1 in, 6 out]
        n205 = local read "Стоп"() -> (w428:bool)
      }
    }
  }
  n206 = while {
    shift-right: [w429] -> _
    shift-left: 0 -> [w431]
    tunnel: w33 -> [_]
    stop <- w435 stop-if-true
    # "Управление Ардуино тумблерами"
    n207 = local read "Стоп"() -> (w435:bool)
    n208 = Boolean Array To Number(Boolean array="Сегменты") -> (number=w430:u32)
    n209 = Wait (ms)(milliseconds to wait=u32 10 ("millisecond timer value")) -> ()  [unwired: 1 out]
    n210 = To Long Integer(number=w430) -> (32bit integer=w429:i32)
    n211 = Not Equal?(x=w429, y=w431) -> (x != y?=w433:bool)
    n212 = case shown="True" w433 {
      tunnel: w429 -> [_ w436]
      tunnel: w431 -> [_ w437]
      frame False {
      }
      frame True {
        n213 = stacked-sequence {
          seq-local: [w440 _ _] -> [_ w445 _]
          seq-local: [w438 _ _] -> [_ w449 _]
          seq-local: [_ w450 _] -> [_ _ w487]
          tunnel: w436 -> [w442 _ _]
          tunnel: w437 -> [w441 _ _]
          frame #0 {
            # "Детектирвоание позиции и\nнаправления изменения бита"
            n214 = Subtract(x=w442, y=w441) -> (x-y=w443:i32)
            n215 = To Double Precision Float(number=w443) -> (double precision float=w444:dbl)
            n216 = Greater Than 0?(x=w443) -> (x > 0?=w440:bool)
            "+/-" <- w440
            n217 = Absolute Value(x=w444) -> (abs(x)=w439:dbl)
            n218 = Logarithm Base 2(1:w439) -> (0:w438:dbl)
            "Разряд" <- w438
          }
          frame #1 {
            # "последний включенный сегмент"
            # "Выбор бита и направления\n его измнения"
            n219 = case shown="10" w449 {
              tunnel: ["D10" "D9" "D5" "D8" "D11" "D12" "A1" "D4" "A5" "A4" "A3" "A2" "A0" "D13" "D3" "All"] -> w447
              tunnel: ["a" "b" "c" "d" "e" "f" "g" "h" "j" "k" "L" "m" "n" "p" "dp" "All"] -> w446
              frame 0, Default {
                # "a = D10"
              }
              frame 1 {
                # "b = D9"
              }
              frame 2 {
                # "c = D5"
              }
              frame 3 {
                # "d = D8"
              }
              frame 4 {
                # "e = D11"
              }
              frame 5 {
                # "f = D12"
              }
              frame 6 {
                # "g = A1"
              }
              frame 7 {
                # "h = D4"
              }
              frame 8 {
                # "j = A5"
              }
              frame 9 {
                # "k = A4"
              }
              frame 10 {
                # "L = A3"
              }
              frame 11 {
                # "m = A2"
              }
              frame 12 {
                # "n = A0"
              }
              frame 13 {
                # "p = D13"
              }
              frame 14 {
                # "dp = D3"
              }
              frame 15 {
              }
            }
            n220 = Select(t="off", s=w445, f="on") -> (s? t:f=w448:string)
            n221 = Concatenate Strings(w447, "_" ("string"), w448) -> (w450:string)
            n222 = case shown="True" w445 {
              tunnel: w446 -> [_ w454]
              frame False {
              }
              frame True {
                "Сегмент" <- w454
              }
            }
          }
          frame #2 {
            # "Передача команды в Ардуино"
            n223 = disable-structure shown="Disabled" {
              disable-tunnel: w487 -> [w489 _]
              frame Disabled {
                n224 = Equal?(x=w489, y="All_off") -> (x = y?=w492:bool)
                n225 = Equal?(x=w489, y="All_on") -> (x = y?=w490:bool)
                n226 = case shown="True" w492 {
                  frame False {
                  }
                  frame True {
                    n227 = local write "Сегменты"(bool[] [TRUE, TRUE, TRUE, TRUE, TRUE, TRUE, TRUE, TRUE, TRUE, TRUE, TRUE, TRUE, TRUE, TRUE, TRUE, TRUE] ("Сегменты")) -> ()
                  }
                }
                n228 = case shown="True" w490 {
                  frame False {
                  }
                  frame True {
                    n229 = local write "Сегменты"(bool[] [FALSE, FALSE, FALSE, FALSE, FALSE, FALSE, FALSE, FALSE, FALSE, FALSE, FALSE, FALSE, FALSE, FALSE, FALSE, FALSE] ("Сегменты")) -> ()
                  }
                }
              }
              frame Enabled {
              }
            }
            n230 = stacked-sequence {
              tunnel: w487 -> [w495 _ _]
              frame #0 {
                n231 = local write "Command"(w495) -> ()
              }
              frame #1 {
                n232 = local write "Записать"(TRUE ("Записать")) -> ()
                n233 = Wait (ms)(milliseconds to wait=u32 1000) -> ()  [unwired: 1 out]
              }
              frame #2 {
                n234 = local write "Записать"(FALSE ("Записать")) -> ()
                n235 = Wait (ms)(milliseconds to wait=u32 1000) -> ()  [unwired: 1 out]
              }
            }
          }
        }
      }
    }
  }
  n236 = call <instrlib>:"niDMM Close.vi"("error in (no error)"=w26, "instrument handle"=w27) -> ()  [unwired: 9 in, 1 out]
  n237 = while {
    tunnel: [w506] -> w28
    tunnel: w31 -> [w504]
    tunnel: w30 -> [w503]
    tunnel: [w500] -> w29
    stop <- w502 stop-if-true
    # "Настройка вольтметра NI PXI-4071"
    n238 = Wait (ms)(milliseconds to wait=u32 1) -> ()  [unwired: 1 out]
    n239 = flat-sequence {
      tunnel: [w513] -> w508
      tunnel: w504 -> [w511]
      tunnel: w503 -> [w515]
      tunnel: [w512] -> w507
      tunnel: w508 -> [w525]
      tunnel: w507 -> [w528]
      tunnel: [w524] -> w502
      tunnel: [w523] -> w500
      tunnel: [w522] -> w501
      frame #0 {
        w509 = T6 6.5 items=["3 1/2"=3.5, "4 1/2"=4.5, "5 1/2"=5.5, "6 1/2"=6.5, "7 1/2"=7.5] ("Resolution in Digits")
        n240 = Fract/Exp String To Number(string="NI DMM 1 Voltage Range 4") -> (number=w514:dbl)  [unwired: 3 in, 1 out]
        n241 = call-poly <instrlib>:"niDMM Config Measurement.vi"("Range"=w514, "Resolution in Digits"=w509, "error in (no error)"=w515, "Function"=niDMM_Function."DC Volts" ("Measurement Type"), "instrument handle"=w511) -> ("error out"=w512:errorcluster, "instrument handle out"=w513:refnum<k15>)  [unwired: 5 in]
      }
      frame #1 {
        n242 = call <instrlib>:"niDMM Read.vi"("error in (no error)"=w528, "instrument handle"=w525) -> ("error out"=w522:errorcluster, "Measurement"=w517:dbl, "instrument handle out"=w523:refnum<k15>)  [unwired: 7 in]
        n243 = Fract/Exp String To Number(string="NI DMM 1 units 4") -> (number=w526:dbl)  [unwired: 3 in, 1 out]
        n244 = Multiply(x=w526, y=w517) -> (x*y=w519:dbl)
        n245 = Absolute Value(x=w519) -> (abs(x)=→"Voltage Char":dbl)
        n246 = Absolute Value(x=w519) -> (abs(x)=→"Voltage":dbl)
        n247 = Absolute Value(x=w517) -> (abs(x)=→"Voltage, V":dbl)
        n248 = local read "Стоп"() -> (w524:bool)
      }
    }
    n249 = call <vilib>:"Simple Error Handler.vi"("error in (no error)"=w501) -> ("error out"=w506:errorcluster)  [unwired: 1 in, 7 out]
  }
  n250 = invoke class="AmateurStepperMotor" method="Stop"(reference=w6) -> (reference out=w13:refnum<k24>, "Stop"=w14:refnum<k24>)  [unwired: 2 in, 1 out]
  n251 = property class="AmateurStepperMotor"(reference=w13, "HoldOn"=FALSE) -> (reference out=w12:refnum<k24>)  [unwired: 1 in, 1 out]
  n252 = invoke class="AmateurStepperMotor" method="Dispose"(reference=w12) -> (error out=w9:errorcluster)  [unwired: 2 in, 2 out]
  n253 = invoke class="SerialPort" method="Close"(reference=w19, error in=w9) -> (reference out=w8:refnum<k24>, error out=w10:errorcluster)  [unwired: 1 in, 1 out]
  n254 = invoke class="Task" method="Wait"(reference=w14) -> ()  [unwired: 2 in, 3 out]
  n255 = Close Reference(reference=w8, error in (no error)=w10) -> (error out=w11:errorcluster)
  n256 = call <vilib>:"Simple Error Handler.vi"("error in (no error)"=w11) -> ()  [unwired: 1 in, 8 out]
  n257 = VISA Close(VISA resource name=w17, error in (no error)=w16) -> (error out=w21:errorcluster)
  n258 = call <instrlib>:"niDMM Close.vi"("error in (no error)"=w28, "instrument handle"=w29) -> ()  [unwired: 9 in, 1 out]
  n259 = call <instrlib>:"niDCPower Close.vi"("instrument handle"=w34) -> ()  [unwired: 10 in, 1 out]
  n260 = call "Ophir Error Message.vi"("error in (no error)"=w21) -> ()  [unwired: 3 in, 4 out]
